vi "_PathQ.vi"(8 "error in (no error)":errorcluster) -> (0 "error out":errorcluster, 3 "Queue out":refnum<queue>)   [LabVIEW 2019, in "LabVIEW-ProviderShell.lvlib" / "VIProviderShellHelper.lvclass"]
uses:
  VIProviderShellHelper.lvclass
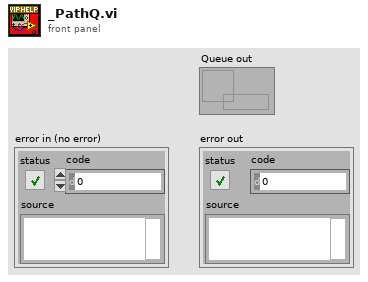
[diagram p1: front panel]
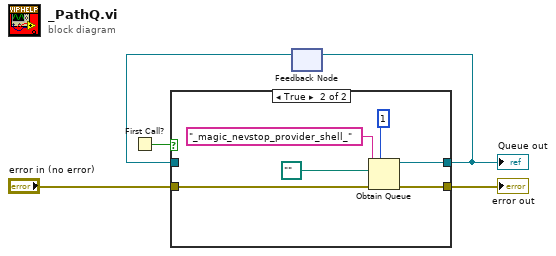
[diagram p0: block diagram]
diagram:
  n1 = First Call?() -> (First Call?: T/F=w3:bool)
  n2 = feedback #1() -> (w5:refnum<queue>)  [unwired: 1 in]
  n3 = case shown="True" w3 {
    tunnel: [w6 w13] -> w1
    tunnel: [w7 w12] -> w4
    tunnel: "error in (no error)" -> [w6 w9]
    tunnel: w5 -> [w7 _]
    frame False {
    }
    frame True {
      n4 = Obtain Queue(max queue size (-1, unlimited)=1, name (unnamed)="_magic_nevstop_provider_shell_", element data type=path "" ("Initialize-API"), error in (no error)=w9) -> (queue out=w12:refnum<queue>, error out=w13:errorcluster)  [unwired: 1 in, 1 out]
    }
  }
  "Queue out" <- w4
  "error out" <- w1
  n5 = feedback-in #1(w4) -> ()
